vi "GDSString_ExtractEnumInfoFromText.vi"(8 "error in (no error)":errorcluster, 11 "AttributeStringIn":string="private int i=0;\npublic static enum Orientation {\n    TOP, LEFT\n  }\n//This is a Range Enum\nenum Range : long { Max = 2147483648L, Min = 255L };\n[Flags]\npublic enum CarOptions\n{\n    // The flag for SunRoof is 0001.\n    SunRoof = 0x01,\n    // The flag for Spoiler is 0010.\n    Spoiler = 0x02,\n    // The flag for FogLights is 0100.\n    FogLights = 0x04,\n    // The flag for TintedWindows is 1000.\n    TintedWindows = 0x08,\n}\n/***\nThis is my struct\n*/\nprivate int x=0;\npublic struct Book\n{\n    public decimal price;\n    public string title;\n    public string author;\n}\n\npublic static enum Orientation {\n    TOP, LEFT\n  }") -> (0 "error out":errorcluster, 1 "Structs":T1[](array[typedef])=[{"Name"="Book", "AccessScope"=enum."public", "Modifiers"=[], "Items"=[{"Name"="", "DataType"=enum."UINT8", "ArrayDim"=0, "CtrlPath"=path "", "DataTypeString"="", "AccessScope"=enum."public", "InitialData"=variant}, {"Name"="", "DataType"=enum."UINT8", "ArrayDim"=0, "CtrlPath"=path "", "DataTypeString"="", "AccessScope"=enum."public", "InitialData"=variant}, {"Name"="", "DataType"=enum."UINT8", "ArrayDim"=0, "CtrlPath"=path "", "DataTypeString"="", "AccessScope"=enum."public", "InitialData"=variant}], "Documentation"=""}], 2 "Enums":T6[](array[typedef])=[{"Name"="Orientation", "AccessScope"=enum."public", "Modifiers"=[], "Items"=["TOP", "LEFT"], "Documentation"=""}, {"Name"="Range", "AccessScope"=enum."public", "Modifiers"=[], "Items"=["Max", "Min"], "Documentation"=""}, {"Name"="CarOptions", "AccessScope"=enum."public", "Modifiers"=[], "Items"=["SunRoof", "Spoiler", "FogLights", "TintedWindows"], "Documentation"=""}], 3 "StructsAndEnumsRemoved":string)   [LabVIEW 2012]
uses:
  <resource>/Framework/Providers/Open_GDS/ClassProviders/Common/CommonVIs/CommonVIs_EnumType.ctl
  <resource>/Framework/Providers/Open_GDS/ClassProviders/Common/String/GDSString_AccessScopeModifierType.ctl
  <resource>/Framework/Providers/Open_GDS/ClassProviders/Common/String/GDSString_ModifierType.ctl
  <resource>/Framework/Providers/Open_GDS/ClassProviders/Common/CommonVIs/CommonVIs_StructType.ctl
  <resource>/Framework/Providers/Open_GDS/ClassProviders/Common/CommonVIs/CommonVIs_AttributeType.ctl
  <resource>/Framework/Providers/Open_GDS/ClassProviders/Common/CommonVIs/CommonVIs_AttributeDataType.ctl
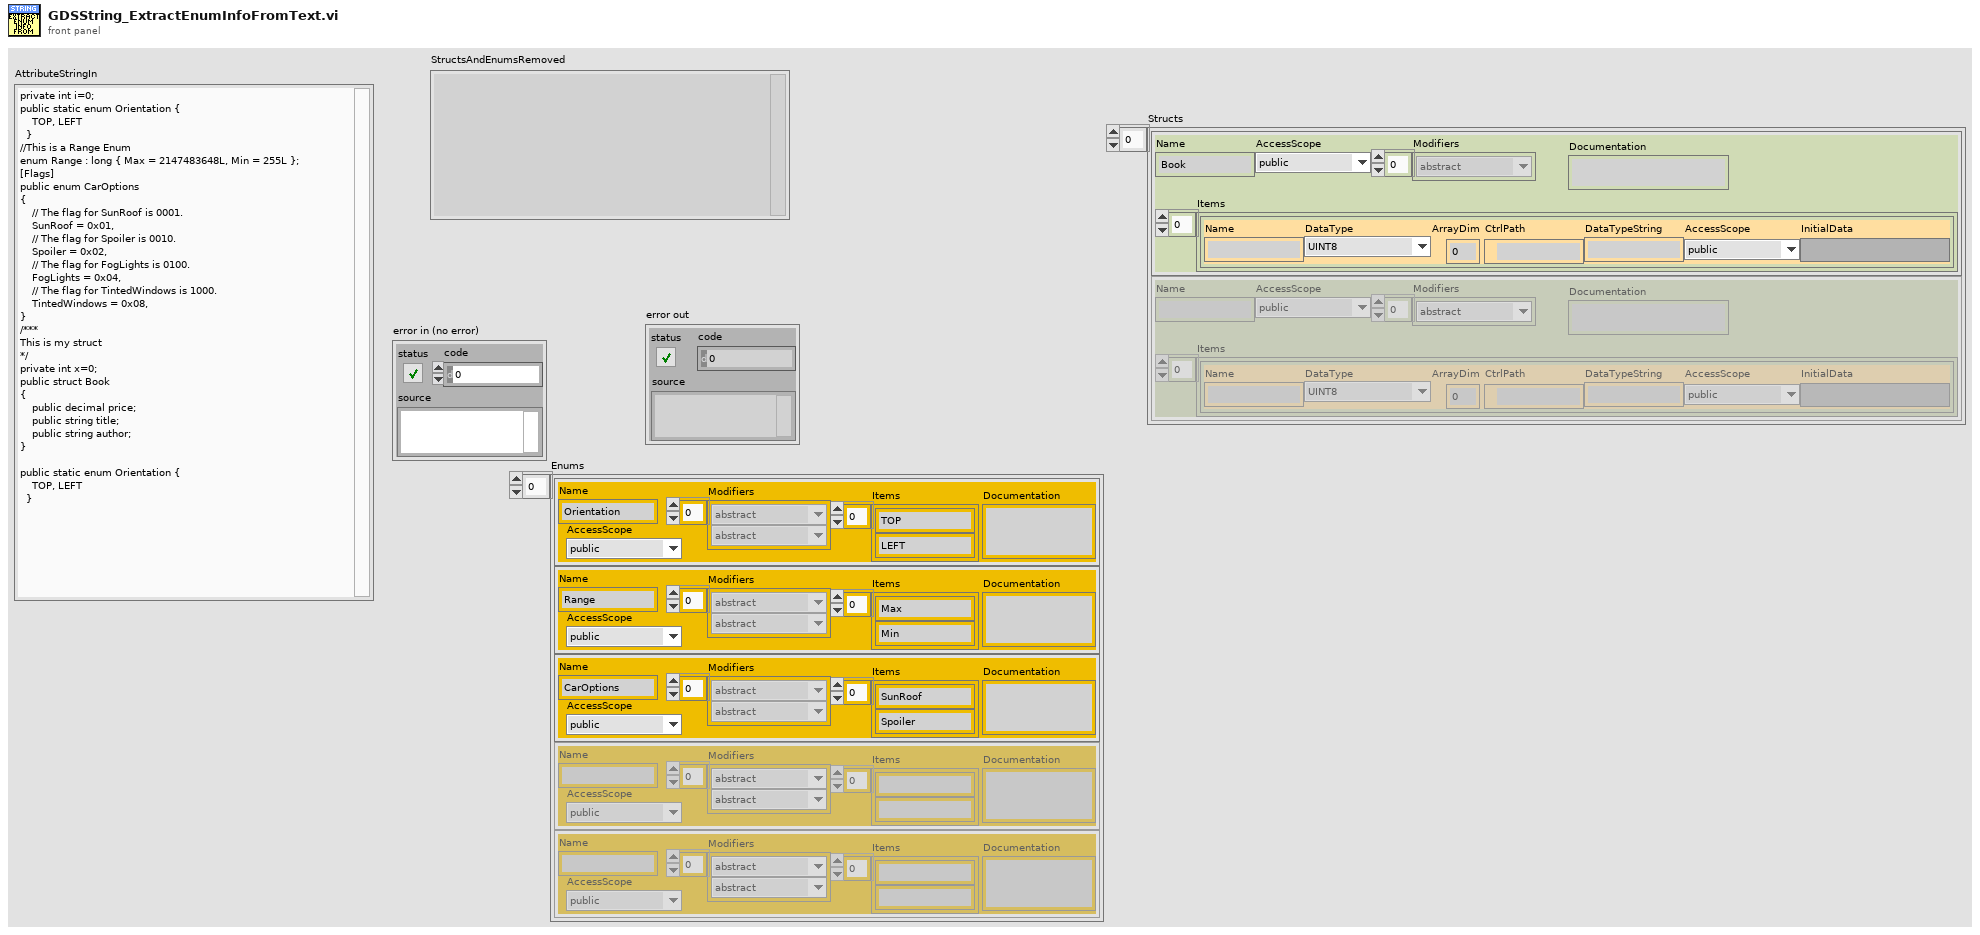
[diagram p1: front panel]
types:
  T1 = typedef "CommonVIs_StructType.ctl" = cluster{"Name":string, "AccessScope":T2, "Modifiers":T3[], "Items":T4[], "Documentation":string}
  T2 = typedef "GDSString_AccessScopeModifierType.ctl" = enum16{"public", "private", "protected", "internal"}
  T3 = typedef "GDSString_ModifierType.ctl" = enum16{"abstract", "static", "final", "synchronized", "strictfp", "async", "const", "event", "extern", "new", "native ", "override", "partial", "readonly", "sealed", "unsafe", "virtual", "volatile"}
  T4 = typedef "CommonVIs_AttributeType.ctl" = cluster{"Name":string, "DataType":T5, "ArrayDim":i32, "CtrlPath":path, "DataTypeString":string, "AccessScope":T2, "InitialData":variant}
  T5 = typedef "CommonVIs_AttributeDataType.ctl" = enum16{"UINT8", "INT8", "UINT16", "INT16", "UINT32", "INT32", "UINT64", "INT64", "SGL", "DBL", "EXT", "CSG", "CDB", "CXT", "TimeStamp", "STRING", "PATH", "BOOL", "ENUM", "RefNum", "VIRefNum", "LabVIEW Class", "Cluster", "Variant", "TypeDef", "Waveform", "LabVIEW Object", "Other", "void"}
  T6 = typedef "CommonVIs_EnumType.ctl" = cluster{"Name":string, "AccessScope":T2, "Modifiers":T3[], "Items":string[], "Documentation":string}
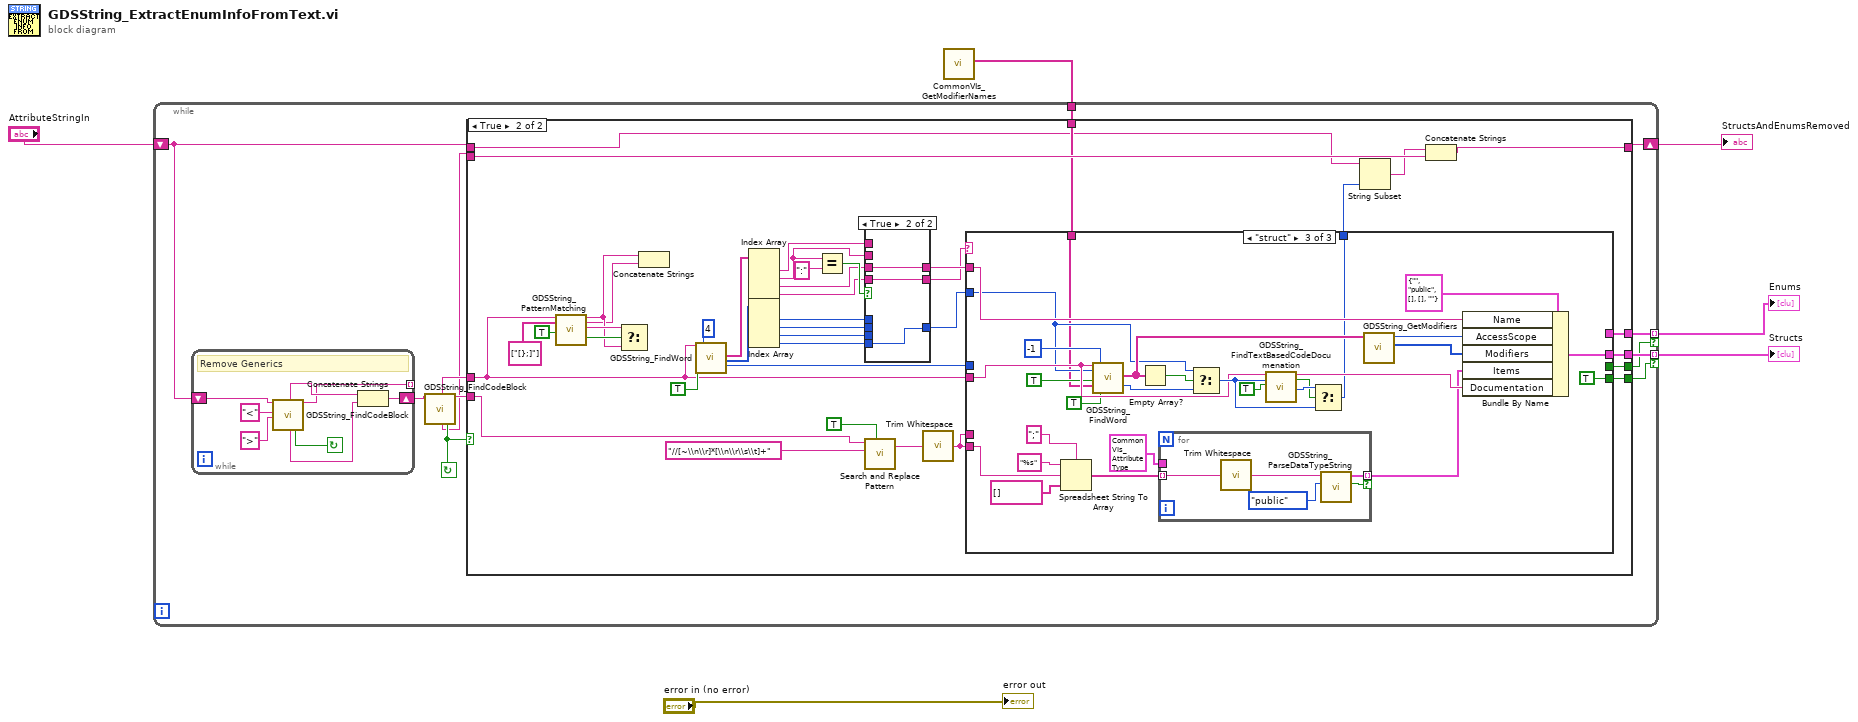
[diagram p0: block diagram]
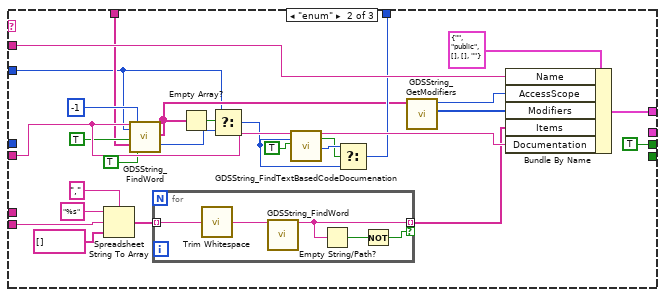
[diagram p5: hidden frame]
diagram:
  n1 = call <resource>:"CommonVIs_GetModifierNames.vi"() -> ("AllModifiers"=w1:string[])  [unwired: 9 in, 2 out]
  n2 = while {
    tunnel: [w16] -> w6 mode=indexing if=w13
    tunnel: [w15] -> w5 mode=indexing if=w14
    shift-right: [w11] -> w2
    shift-left: "AttributeStringIn" -> [w8]
    tunnel: w1 -> [w9]
    stop <- w12 continue-if-true
    n3 = while {
      shift-right: [w20] -> w7
      shift-left: w8 -> [w26]
      tunnel: [w19] -> _ mode=indexing
      stop <- w23 continue-if-true
      # "Remove Generics"
      n4 = call <resource>:"GDSString_FindCodeBlock.vi"("Text"=w26, "CodeBlockStartCharacter( { )"="<", "CodeBlockEndCharacter( } )"=">") -> ("TextBeforeBlock"=w22:string, "TextAfterBlock"=w21:string, "found"=w23:bool, "BlockText"=w19:string)  [unwired: 8 in, 5 out]
      n5 = Concatenate Strings(w22, w21) -> (w20:string)
    }
    n6 = call <resource>:"GDSString_FindCodeBlock.vi"("Text"=w7) -> ("TextBeforeBlock"=w18:string, "TextAfterBlock"=w10:string, "found"=w12:bool, "BlockText"=w17:string)  [unwired: 10 in, 5 out]
    n7 = case shown="True" w12 {
      tunnel: w18 -> [_ w32]
      tunnel: w17 -> [_ w52]
      tunnel: [_ w63] -> w16
      tunnel: [_ w49] -> w15
      tunnel: [_ w48] -> w14
      tunnel: [_ w47] -> w13
      tunnel: w8 -> [w27 w31]
      tunnel: [w27 w28] -> w11
      tunnel: w10 -> [_ w40]
      tunnel: w9 -> [_ w33]
      frame False {
      }
      frame True {
        n8 = call <resource>:"GDSString_PatternMatching.vi"("TextIn"=w32, "PatternMatchingStrings"=string[] ["[};]"] ("PatternMatchingString"), "Search Backwards"=TRUE) -> ("TextBefore"=w42:string, "Match"=w41:string, "TextAfter"=w43:string, "Found"=w44:bool)  [unwired: 10 in, 3 out]
        n9 = Select(t=w43, s=w44, f=w42) -> ()  [unwired: 1 out]
        n10 = Concatenate Strings(w42, w41) -> ()  [unwired: 1 out]
        n11 = call <resource>:"GDSString_FindWord.vi"("Text"=w32, "Search Backwards"=TRUE, "GetNext-X_Words(1,-1=All)"=4 ("GetNext-X_Words(1)")) -> ("NextWords"=w65:string[], "IndexAfterMatches(Or before when searching Backwards)"=w39:i32[], "IndexAfterLastMatch(Or before when searching Backwards)"=w64:i32)  [unwired: 11 in, 3 out]
        n12 = Index Array(array=w65) -> (element #1=w60:string, element #2=w58:string, element #3=w56:string, element #4=w55:string)  [unwired: 4 in]
        n13 = Index Array(array=w39) -> (element #1=w38:i32, element #2=w37:i32, element #3=w34:i32, element #4=w35:i32)  [unwired: 4 in]
        n14 = Equal?(x=w58, y=":") -> (x = y?=w61:bool)
        n15 = case shown="True" w61 {
          tunnel: w60 -> [w70 _]
          tunnel: [w70 w73] -> w59
          tunnel: w58 -> [w69 _]
          tunnel: [w69 w72] -> w57
          tunnel: w56 -> [_ w73]
          tunnel: w55 -> [_ w72]
          tunnel: w38 -> [_ _]
          tunnel: w37 -> [w68 _]
          tunnel: [w68 w71] -> w36
          tunnel: w35 -> [_ w71]
          tunnel: w34 -> [_ _]
          frame False {
          }
          frame True {
          }
        }
        n16 = call <vilib>:"Search and Replace Pattern.vi"("string"=w52, "regular expression (\"\")"="//[~\\n\\r]*[\\n\\r\\s\\t]+" ("regular expression (\"\")"), "replace all? (F)"=TRUE) -> ("result string"=w51:string)  [unwired: 2 in, 1 out]
        n17 = call <vilib>:"Trim Whitespace.vi"("string"=w51) -> ("trimmed string"=w50:string)  [unwired: 1 in]
        n18 = case shown="\"struct\"" w57 {
          tunnel: w59 -> [_ w100 w133]
          tunnel: w32 -> [_ w95 w125]
          tunnel: w64 -> [_ _ _]
          tunnel: w50 -> [_ w92 w122]
          tunnel: [_ w86 _] -> w63
          tunnel: w50 -> [_ _ _]
          tunnel: [_ _ w117] -> w49
          tunnel: [_ _ TRUE] -> w48
          tunnel: [_ TRUE _] -> w47
          tunnel: w36 -> [_ w77 w109]
          tunnel: w33 -> [_ w81 w108]
          tunnel: [_ w80 w107] -> w30
          frame Default {
          }
          frame "enum" {
            n19 = Spreadsheet String To Array(delimiter (Tab)=",", format string="%s", spreadsheet string=w92, array type (2D Dbl)=string[] []) -> (array=w88:string[])
            n20 = call <resource>:"GDSString_FindWord.vi"("Text"=w95, "StringStartOffset(Default=-1 => 0 for Forward, StrLenght for Backwards)"=w77, "Search Backwards"=TRUE, "AllowedWords(PatternMatching)"=w81, "GetNext-X_Words(1,-1=All)"=-1, "ExactWord"=TRUE) -> ("NextWords"=w78:string[], "IndexAfterLastMatch(Or before when searching Backwards)"=w76:i32)  [unwired: 8 in, 4 out]
            n21 = for {
              tunnel: w88 -> [w105] mode=indexing
              tunnel: [w103] -> w87 mode=indexing if=w101
              n22 = call <vilib>:"Trim Whitespace.vi"("string"=w105) -> ("trimmed string"=w104:string)  [unwired: 1 in]
              n23 = call <resource>:"GDSString_FindWord.vi"("Text"=w104) -> ("NextWord"=w103:string)  [unwired: 13 in, 5 out]
              n24 = Empty String/Path?(string/path=w103) -> (empty?=w102:bool)
              n25 = Not(x=w102) -> (.not. x?=w101:bool)
            }
            n26 = Empty Array?(array=w78) -> (empty?=w79:bool)
            n27 = Select(t=w77, s=w79, f=w76) -> (s? t:f=w75:i32)
            n28 = call <resource>:"GDSString_FindTextBasedCodeDocumenation.vi"("Text"=w95, "StringStartOffset(Default=-1 => 0 for Forward, StrLenght for Backwards)"=w75, "Search Backwards"=TRUE) -> ("Document"=w93:string, "Found"=w98:bool, "IndexBeforeDocument(Or after when searching Backwards)"=w99:i32)  [unwired: 12 in, 2 out]
            n29 = Select(t=w99, s=w98, f=w75) -> (s? t:f=w80:i32)
            n30 = call <resource>:"GDSString_GetModifiers.vi"("Words"=w78) -> ("Array out"=w83:T3[], "AccessScope"=w84:T2)  [unwired: 8 in, 1 out]
            n31 = Bundle By Name(cluster=T6 {"Name"="", "AccessScope"=enum."public", "Modifiers"=[], "Items"=[], "Documentation"=""} ("EnumType"), "Name"=w100, "AccessScope"=w84, "Modifiers"=w83, "Items"=w87, "Documentation"=w93) -> (w86:T6)
          }
          frame "struct" {
            n32 = Spreadsheet String To Array(delimiter (Tab)=";", format string="%s", spreadsheet string=w122, array type (2D Dbl)=string[] []) -> (array=w118:string[])
            n33 = call <resource>:"GDSString_FindWord.vi"("Text"=w125, "StringStartOffset(Default=-1 => 0 for Forward, StrLenght for Backwards)"=w109, "Search Backwards"=TRUE, "AllowedWords(PatternMatching)"=w108, "GetNext-X_Words(1,-1=All)"=-1, "ExactWord"=TRUE) -> ("NextWords"=w113:string[], "IndexAfterLastMatch(Or before when searching Backwards)"=w129:i32)  [unwired: 8 in, 4 out]
            n34 = Empty Array?(array=w113) -> (empty?=w128:bool)
            n35 = for {
              tunnel: w118 -> [w138] mode=indexing
              tunnel: [w135] -> w110 mode=indexing if=w134
              tunnel: T4 {"Name"="", "DataType"=enum."UINT8", "ArrayDim"=0, "CtrlPath"=path "", "DataTypeString"="", "AccessScope"=enum."public", "InitialData"=variant} ("DataType") -> [_]
              n36 = call <vilib>:"Trim Whitespace.vi"("string"=w138) -> ("trimmed string"=w137:string)  [unwired: 1 in]
              n37 = call <resource>:"GDSString_ParseDataTypeString.vi"("DefaultAccessScope(Private)"=GDSString_AccessScopeModifierType."public", "InputText"=w137) -> ("Found"=w134:bool, "DataType"=w135:T4)  [unwired: 7 in, 1 out]
            }
            n38 = Select(t=w109, s=w128, f=w129) -> (s? t:f=w132:i32)
            n39 = call <resource>:"GDSString_FindTextBasedCodeDocumenation.vi"("Text"=w125, "StringStartOffset(Default=-1 => 0 for Forward, StrLenght for Backwards)"=w132, "Search Backwards"=TRUE) -> ("Document"=w123:string, "Found"=w130:bool, "IndexBeforeDocument(Or after when searching Backwards)"=w131:i32)  [unwired: 12 in, 2 out]
            n40 = Select(t=w131, s=w130, f=w132) -> (s? t:f=w107:i32)
            n41 = call <resource>:"GDSString_GetModifiers.vi"("Words"=w113) -> ("Array out"=w114:T3[], "AccessScope"=w115:T2)  [unwired: 8 in, 1 out]
            n42 = Bundle By Name(cluster=T1 {"Name"="", "AccessScope"=enum."public", "Modifiers"=[], "Items"=[], "Documentation"=""} ("StructType"), "Name"=w133, "AccessScope"=w115, "Modifiers"=w114, "Items"=w110, "Documentation"=w123) -> (w117:T1)
          }
        }
        n43 = String Subset(string=w31, length (rest)=w30) -> (substring=w29:string)  [unwired: 1 in]
        n44 = Concatenate Strings(w29, w40) -> (w28:string)
      }
    }
  }
  "Enums" <- w6
  "Structs" <- w5
  "StructsAndEnumsRemoved" <- w2
  "error out" <- "error in (no error)"
